vi "Configure Data Logging.vi"(8 "error in (no error)":errorcluster, 9 "Interval (10)":dbl=10.0, 10 "Logging Type (0: Internal)":u16(ring) items=["Internal", "External"], 11 "VISA resource name":refnum<visa-resource-name>) -> (0 "error out":errorcluster, 3 "VISA resource name out":refnum<visa-resource-name>)   [LabVIEW 2013, in "Watts Up Series.lvlib"]
doc: "Configure the <b>logging type</b> and the <b>interval rate</b> of the data capture for the Watts Up device."
uses:
  <instrlib>/Watts Up Series/Watts Up Series.lvlib
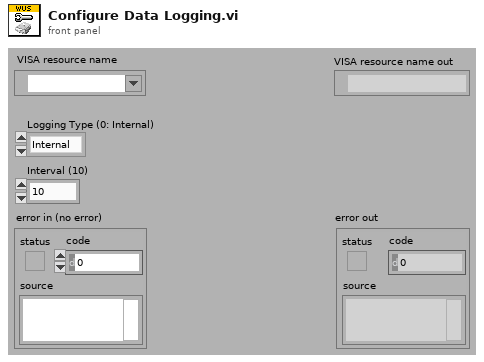
[diagram p1: front panel]
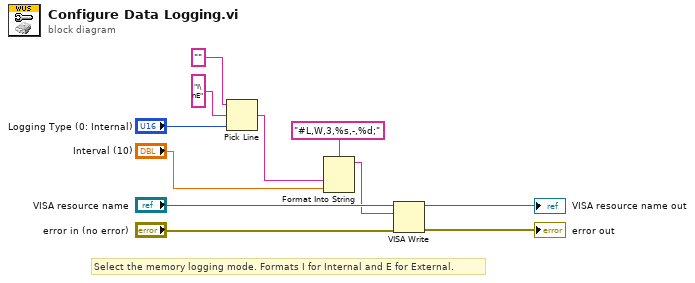
[diagram p0: block diagram]
diagram:
  # "Select the memory logging mode. Formats I for Internal and E for External."
  n1 = Pick Line(string ("")="", multi-line string="I\nE", line index="Logging Type (0: Internal)") -> (output string=w3:string)
  n2 = Format Into String(format string="#L,W,3,%s,-,%d;", w3, "Interval (10)") -> (resulting string=w1:string)  [unwired: 2 in, 1 out]
  n3 = VISA Write(VISA resource name="VISA resource name", write buffer=w1, error in (no error)="error in (no error)") -> (VISA resource name out=→"VISA resource name out":refnum<visa-resource-name>, error out=→"error out":errorcluster)  [unwired: 1 out]
